vi "Acquire Image.vi"(8 "error in (no error)":errorcluster, 10 "Readout Timeout":i64=2000, 11 "Picam in":refnum<class "Picam.lvclass">) -> (0 "error out":errorcluster, 3 "Picam out":refnum<class "Picam.lvclass">)   [LabVIEW 2019, in "Picam.lvclass"]
doc: "Acquire a single image. Use the Get Image VI to retrieve the data."
uses:
  Picam.lvclass
  Picam.lvclass/Picam.ctl
  picam32_LabView_SDK/PICam_lib/PICam.lvlib
panel:
  out "readout_count":i64
  out "initial_readout":u64
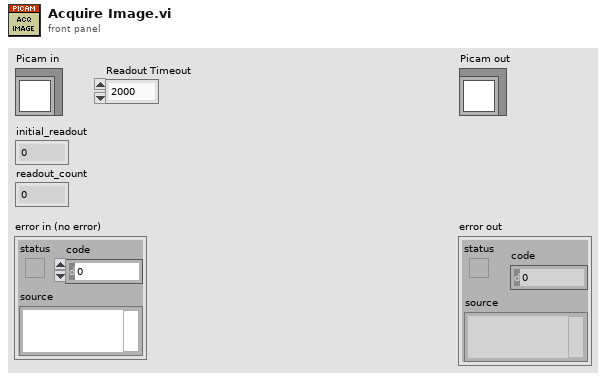
[diagram p1: front panel]
types:
  T1 = typedef "PICam.lvlib/PicamAvailableData.ctl" = cluster{"initial_readout":u64, "readout_count":i64}
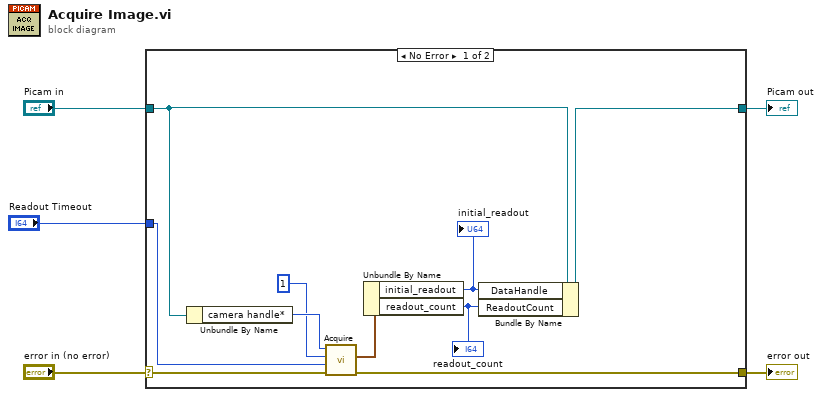
[diagram p0: block diagram]
diagram:
  n1 = case shown="No Error" "error in (no error)" {
    selector: "error in (no error)" -> [w15 w17]
    tunnel: [w14 w17] -> w4
    tunnel: [w10 w16] -> w2
    tunnel: "Picam in" -> [w13 w16]
    tunnel: "Readout Timeout" -> [w6 _]
    frame No Error {
      n2 = Unbundle By Name(w13) -> ("camera handle*"=w12:u64)
      n3 = call "Acquire.vi"("error in (no error)"=w15, "piint (readout_time_out)"=w6, "readout_count"=i64 1, "camera handle in"=w12) -> ("error out"=w14:errorcluster, "PicamAvailableData* (available)"=w9:T1)  [unwired: 4 in, 2 out]
      n4 = Unbundle By Name(w9) -> ("initial_readout"=w8:u64, "readout_count"=w7:i64)
      "initial_readout" <- w8
      "readout_count" <- w7
      n5 = Bundle By Name(cluster=w13, "DataHandle"=w8, "ReadoutCount"=w7) -> (w10:refnum<class "Picam.lvclass">)
    }
    frame Error {
    }
  }
  "error out" <- w4
  "Picam out" <- w2
